vi "Windows.UpdateTime.vi"(8 "error in (no error)":errorcluster, 11 "cmdtime path":path) -> (0 "error out":errorcluster, 2 "cmdtime info":string[](array[string]))   [LabVIEW 2019, in "Tools.lvlib"]
doc: "Update windows local time with the network time servers\n- use 3rd party freeware application (cmdtime)\n- store its events to log them in application event logger\n\nAll hosts connected to Jahont Server should have the same local time for results comparison"
uses:
  Tools.lvlib
panel:
  out "standard output":string
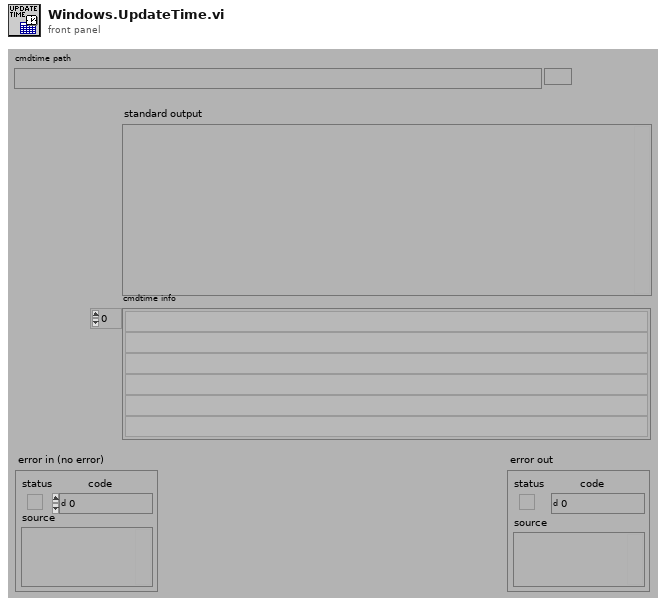
[diagram p1: front panel]
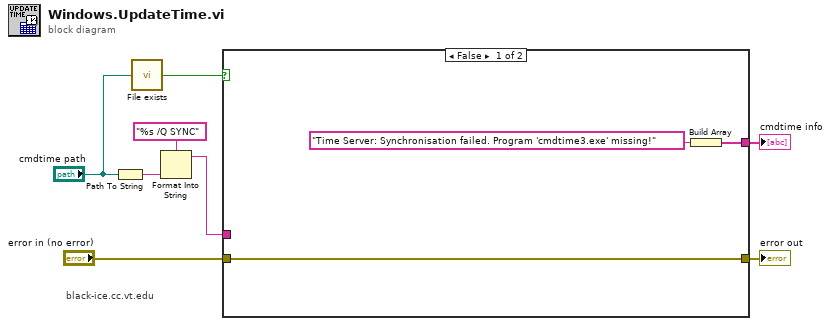
[diagram p0: block diagram]
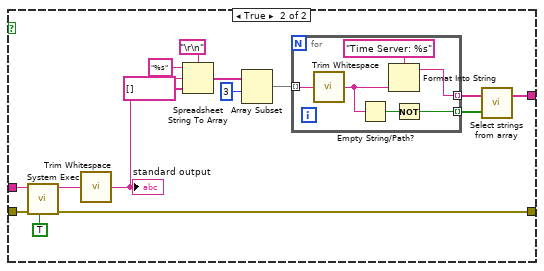
[diagram p2: hidden frame]
diagram:
  # "black-ice.cc.vt.edu"
  n1 = Path To String(path="cmdtime path") -> (string=w6:string)
  n2 = call "File exists.vi"("file path"="cmdtime path") -> ("exists?"=w1:bool)  [unwired: 4 in]
  n3 = Format Into String(format string="%s /Q SYNC", w6) -> (resulting string=w5:string)  [unwired: 2 in, 1 out]
  n4 = case shown="False" w1 {
    tunnel: "error in (no error)" -> [w9 w26]
    tunnel: [w9 w25] -> w7
    tunnel: w5 -> [_ w24]
    tunnel: [w10 w16] -> w3
    frame False {
      n5 = Build Array("Time Server: Synchronisation failed. Program 'cmdtime3.exe' missing!" ("explanation")) -> (w10:string[])
    }
    frame True {
      n6 = call <vilib>:"System Exec.vi"("run minimized? (F)"=TRUE, "error in (no error)"=w26, "command line"=w24) -> ("error out"=w25:errorcluster, "standard output"=w23:string)  [unwired: 5 in, 2 out]
      n7 = call <vilib>:"Trim Whitespace.vi"("string"=w23) -> ("trimmed string"=w19:string)  [unwired: 1 in]
      "standard output" <- w19
      n8 = Spreadsheet String To Array(delimiter (Tab)="\r\n", format string="%s", spreadsheet string=w19, array type (2D Dbl)=string[] []) -> (array=w15:string[])
      n9 = Array Subset(array=w15, index=3) -> (w13:string[])  [unwired: 1 in]
      n10 = for {
        tunnel: w13 -> [w32] mode=indexing
        tunnel: [w30] -> w18 mode=indexing
        tunnel: [w27] -> w17 mode=indexing
        n11 = call <vilib>:"Trim Whitespace.vi"("string"=w32) -> ("trimmed string"=w29:string)  [unwired: 1 in]
        n12 = Empty String/Path?(string/path=w29) -> (empty?=w31:bool)
        n13 = Format Into String(format string="Time Server: %s", w29) -> (resulting string=w27:string)  [unwired: 2 in, 1 out]
        n14 = Not(x=w31) -> (.not. x?=w30:bool)
      }
      n15 = call "Select strings from array.vi"("selection array"=w18, "strings"=w17) -> ("selected strings"=w16:string[])  [unwired: 1 in]
    }
  }
  "error out" <- w7
  "cmdtime info" <- w3
